vi "Pic Write Img.vi"(8 "error in (no error)":errorcluster, 10 "Picture":picture, 11 "Main Panel in":refnum<class "Main Panel.lvclass">) -> (0 "error out":errorcluster, 3 "Main Panel out":refnum<class "Main Panel.lvclass">)   [LabVIEW 2018, in "Main Panel.lvlib" / "Main Panel.lvclass"]
uses:
  Main Panel.lvclass
  Main Panel.lvclass/Main Panel.ctl
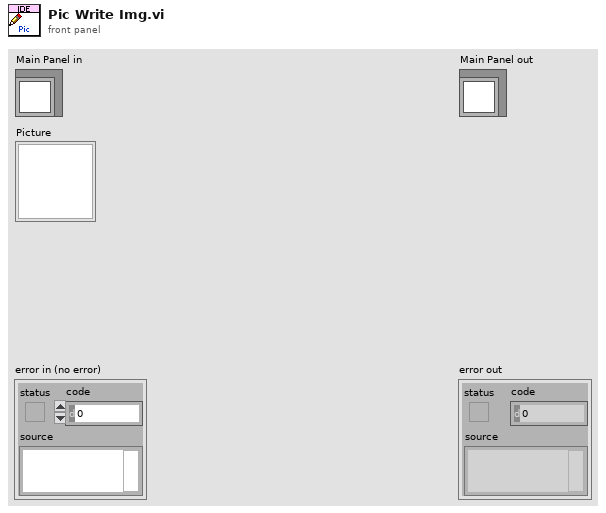
[diagram p1: front panel]
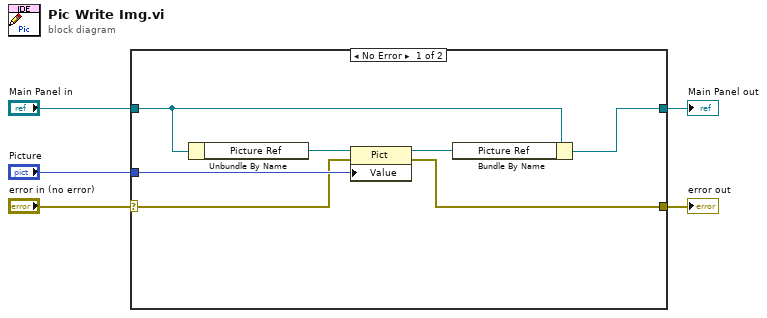
[diagram p0: block diagram]
diagram:
  n1 = case shown="No Error" "error in (no error)" {
    selector: "error in (no error)" -> [w9 w14]
    tunnel: [w8 w14] -> w4
    tunnel: [w7 w13] -> w2
    tunnel: "Main Panel in" -> [w12 w13]
    tunnel: "Picture" -> [w10 _]
    frame No Error {
      n2 = Unbundle By Name(w12) -> ("Picture Ref"=w11:refnum<vi>)
      n3 = property class="Pict"(reference=w11, error in=w9, "Value"=w10) -> (reference out=w6:refnum<vi>, error out=w8:errorcluster)
      n4 = Bundle By Name(cluster=w12, "Picture Ref"=w6) -> (w7:refnum<class "Main Panel.lvclass">)
    }
    frame Error {
    }
  }
  "error out" <- w4
  "Main Panel out" <- w2
